vi "1420sub.vi"(4 "Termination Character":u8=10 format="%.0x", 5 "End Write on Termination Character?":bool=TRUE, 6 "Assert DTR?":bool, 7 "End Read on Termination Character?":bool=TRUE, 8 "Serial Settings":T1={"baud rate"=9600, "data bits"=8, "parity"=enum."None", "stop bits"=10, "flow control"=0} {"flow control" items=["None"=0, "XON/XOFF"=1, "RTS/CTS"=2, "DTR/DSR"=4]; "stop bits" items=["1.0"=10, "1.5"=15, "2.0"=20]; "data bits" min=5 max=8 step=1; "baud rate" items=["75"=75, "110"=110, "134"=134, "150"=150, "300"=300, "600"=600, "1200"=1200, "1800"=1800, "2400"=2400, "4800"=4800, "7200"=7200, "9600"=9600, "14400"=14400, "19200"=19200, "28800"=28800, "38400"=38400, "56000"=56000, "57600"=57600, "115200"=115200, "128000"=128000, "230400"=230400]}, 9 "Write String":string="*IDN?", 10 "stop":bool, 11 "VISA Refnum in":refnum<visa-resource-name>="COM1") -> (3 "x*y":dbl)   [LabVIEW 2019]
uses:
  Program Files (x86)/National Instruments/LabVIEW 2019/examples/Instrument IO/Serial/support/Serial - Settings.ctl
  <vilib>/Instr/_visa.llb/VISA Configure Serial Port (Instr).vi
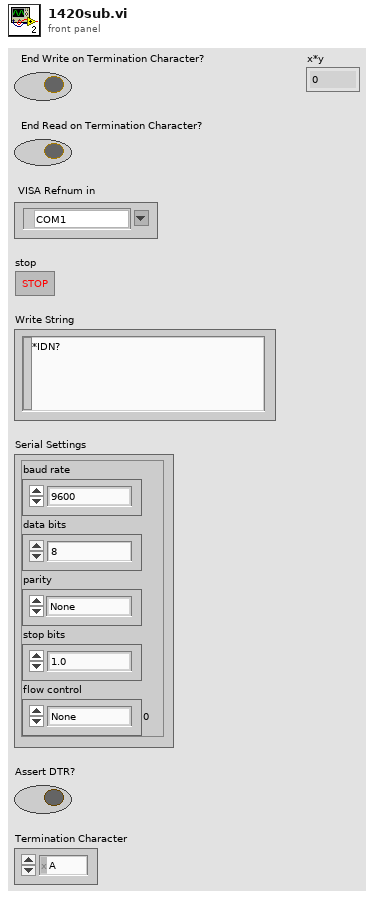
[diagram p1: front panel]
types:
  T1 = typedef "Serial - Settings.ctl" = cluster{"baud rate":u32, "data bits":u16, "parity":enum16{"None", "Odd", "Even", "Mark", "Space"}, "stop bits":u16, "flow control":u16}
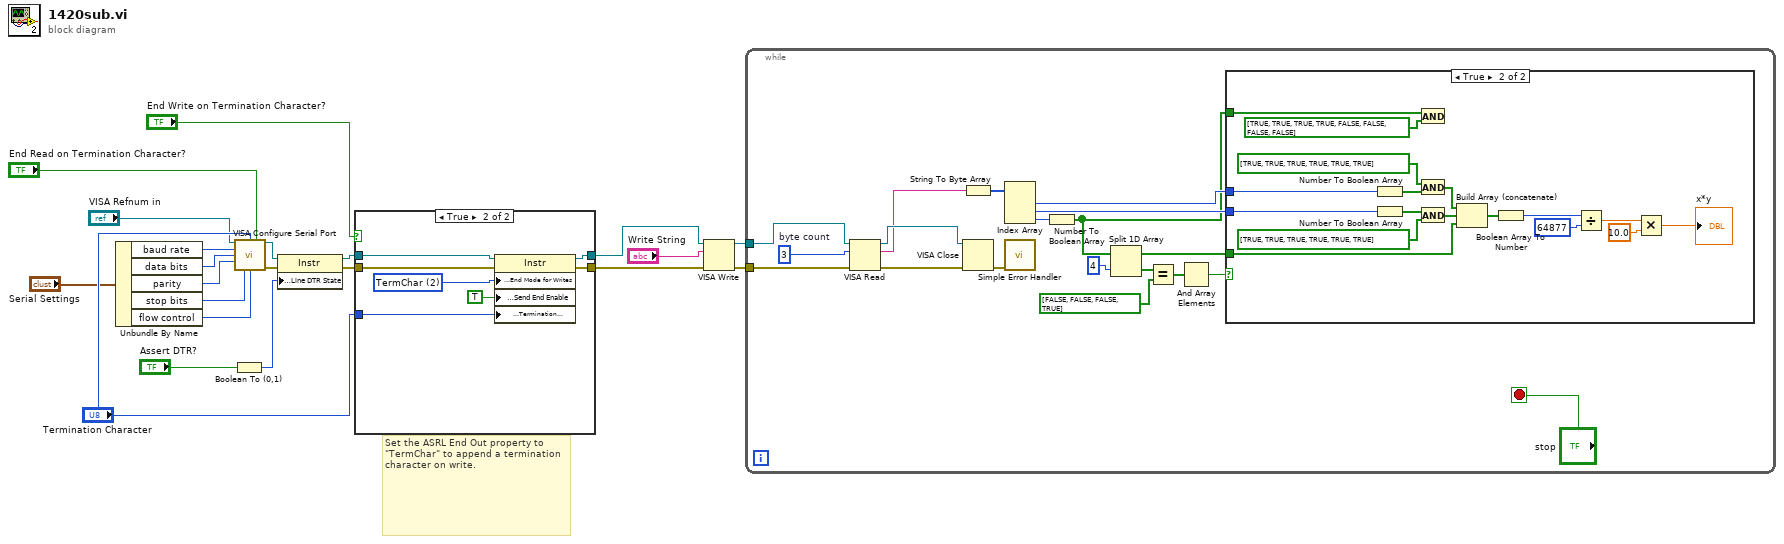
[diagram p0: block diagram]
diagram:
  # "Set the ASRL End Out property to \"TermChar\" to append a termination character on write."
  n1 = Unbundle By Name("Serial Settings") -> ("baud rate"=w9:u32, "data bits"=w10:u16, "parity"=w11:enum16{"None", "Odd", "Even", "Mark", "Space"}, "stop bits"=w12:u16, "flow control"=w13:u16)
  n2 = Boolean To (0,1)(Boolean="Assert DTR?") -> (0, 1=w6:i16)
  n3 = call-poly "VISA Configure Serial Port"("VISA resource name"="VISA Refnum in", "termination char\n(0xA = '\\n' = LF)"="Termination Character", "Enable Termination\nChar (T)"="End Read on Termination Character?", "baud rate (921600)"=w9, "data bits (8)"=w10, "parity (0:none)"=w11, "stop bits (10: 1 bit)"=w12, "flow control (0:none)"=w13) -> ("VISA resource name out"=w3:refnum<visa-resource-name>, "error out"=w4:errorcluster)  [unwired: 2 in, 4 out]
  n4 = property class="Instr"(reference=w3, error in=w4, "Serial Settings:Modem Line Settings:Line DTR State"=w6) -> (reference out=w18:refnum<visa-resource-name>, error out=w17:errorcluster)
  n5 = case shown="True" "End Write on Termination Character?" {
    tunnel: w18 -> [w22 w30]
    tunnel: w17 -> [w23 w29]
    tunnel: [w22 w28] -> w19
    tunnel: [w23 w27] -> w16
    tunnel: "Termination Character" -> [_ w25]
    frame False {
    }
    frame True {
      w26 = u16 2 items=["None", "LastBit", "TermChar", "Break"] ("Serial Settings:Serial End Mode for Writes")
      n6 = property class="Instr"(reference=w30, error in=w29, "Serial Settings:End Mode for Writes"=w26, "Message Based Settings:Send End Enable"=TRUE, "Message Based Settings:Termination Character"=w25) -> (reference out=w28:refnum<visa-resource-name>, error out=w27:errorcluster)
    }
  }
  n7 = VISA Write(VISA resource name=w19, write buffer="Write String", error in (no error)=w16) -> (VISA resource name out=w2:refnum<visa-resource-name>, error out=w7:errorcluster)  [unwired: 1 out]
  n8 = while {
    tunnel: w2 -> [w49]
    tunnel: w7 -> [w46]
    stop <- "stop" stop-if-true
    w44 = u32 3  # byte count
    n9 = VISA Read(VISA resource name=w49, byte count=w44, error in (no error)=w46) -> (VISA resource name out=w47:refnum<visa-resource-name>, read buffer=w43:string, error out=w48:errorcluster)  [unwired: 1 out]
    n10 = String To Byte Array(string=w43) -> (unsigned byte array=w42:u8[])
    n11 = VISA Close(VISA resource name=w47, error in (no error)=w48) -> (error out=w45:errorcluster)
    n12 = Index Array(array=w42) -> (element #1=w41:u8, element #2=w40:u8, element #3=w39:u8)  [unwired: 3 in]
    n13 = call <vilib>:"Simple Error Handler.vi"("error in (no error)"=w45) -> ()  [unwired: 1 in, 8 out]
    n14 = Number To Boolean Array(number=w39) -> (Boolean array=w37:bool[])
    n15 = Split 1D Array(array=w37, index=4) -> (first subarray=w31:bool[], second subarray=w32:bool[])
    n16 = Equal?(x=w32, y=bool[] [FALSE, FALSE, FALSE, TRUE]) -> (x = y?=w33:bool[])
    n17 = And Array Elements(Boolean array=w33) -> (logical AND=w34:bool)
    n18 = case shown="True" w34 {
      tunnel: w41 -> [_ w66]
      tunnel: w40 -> [_ w64]
      tunnel: w37 -> [_ w52]
      tunnel: w31 -> [_ w51]
      frame False {
      }
      frame True {
        n19 = Number To Boolean Array(number=w66) -> (Boolean array=w53:bool[])
        n20 = Number To Boolean Array(number=w64) -> (Boolean array=w63:bool[])
        n21 = And(x=w52, y=bool[] [TRUE, TRUE, TRUE, TRUE, FALSE, FALSE, FALSE, FALSE] ("x")) -> ()  [unwired: 1 out]
        n22 = And(x=bool[] [TRUE, TRUE, TRUE, TRUE, TRUE, TRUE], y=w53) -> (x .and. y?=w54:bool[])
        n23 = And(x=w63, y=bool[] [TRUE, TRUE, TRUE, TRUE, TRUE, TRUE] ("x")) -> (x .and. y?=w55:bool[])
        n24 = Build Array (concatenate)(w54, w55, w51) -> (w60:bool[])
        n25 = Boolean Array To Number(Boolean array=w60) -> (number=w59:u32)
        n26 = Divide(x=w59, y=u32 64877) -> (x/y=w57:dbl)
        n27 = Multiply(x=w57, y=10.0) -> (x*y=→"x*y":dbl)
      }
    }
  }
